vi "PolarNoGrid.vi"(0 "picture":picture, 5 "data array [mag, phase (deg)]":cluster{"magnitude":dbl, "phase":dbl}[](array[cluster]) {"phase" format="%0.2f"; "magnitude" format="%0.2f"}, 7 "top left point(0, 0)":cluster{"x":i16, "y":i16}, 9 "dimensions (w,h)":cluster{"width":i16, "height":i16}, 11 "polar attributes":T1={"maximum"=0.0, "minimum"=0.0, "clip to min"=FALSE, "log?(F)"=FALSE, "grid color"=6710886, "plot color"=65280, "fmt and prec"={"format"=enum."Decimal", "precision"=0}, "visible section"=8} {"minimum" format="%0.2f"; "maximum" format="%0.2f"}, 12 "Lines/Points":enum16{"Lines", "Points"}(ring), 13 "Size":u16=1) -> (4 "new picture":picture)   [LabVIEW 2014]
panel:
  in  "desired font(Application)":T2(ring)=enum."Application Font"
  in  "[user-specified font]":T3
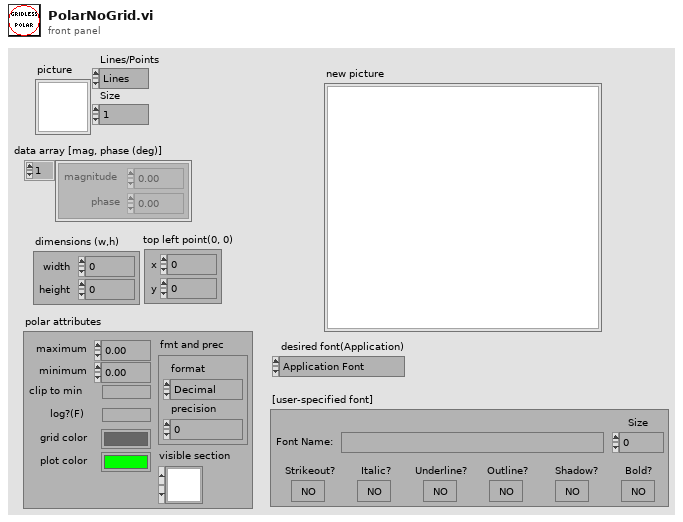
[diagram p1: front panel]
types:
  T1 = cluster{"maximum":dbl, "minimum":dbl, "clip to min":bool, "log?(F)":bool, "grid color":u32, "plot color":u32, "fmt and prec":cluster{"format":enum8{"Decimal", "Scientific", "Engineering", "Binary", "Octal", "Hex"}, "precision":u8}, "visible section":u16}
  T2 = enum16{"User-specified Font", "Application Font", "System Font", "Dialog Font"}
  T3 = cluster{"Font Name:":string, "Size":i16, "Strikeout?":bool, "Italic?":bool, "Underline?":bool, "Outline?":bool, "Shadow?":bool, "Bold?":bool}
  T4 = cluster{"left":i16, "top":i16, "right":i16, "bottom":i16}
  T5 = cluster{"pixel center":cluster{"x":i16, "y":i16}, "scale factors":cluster{"a":dbl, "b":dbl, "log?(F)":bool}, "grid color":u32, "start angle":dbl, "end angle":dbl, "tick length":i16, "pixel radius":i32}
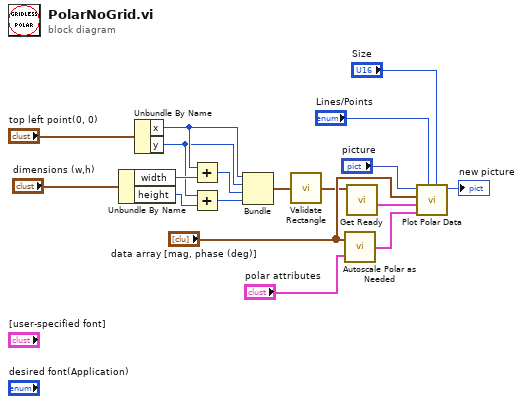
[diagram p0: block diagram]
diagram:
  n1 = Unbundle By Name("dimensions (w,h)") -> ("width"=w12:i16, "height"=w11:i16)
  n2 = Unbundle By Name("top left point(0, 0)") -> ("x"=w10:i16, "y"=w9:i16)
  n3 = Add(x=w10, y=w12) -> (x+y=w8:i16)
  n4 = Add(x=w9, y=w11) -> (x+y=w7:i16)
  n5 = Bundle("x"=w10, "y"=w9, w8, w7) -> (w6:cluster{"x":i16, "y":i16, i16, i16})  [unwired: 1 in]
  n6 = call <vilib>:"Validate Rectangle.vi"("rect"=w6) -> ("valid rect"=w3:T4)
  n7 = call <vilib>:"Autoscale Polar as Needed.vi"("polar attributes"="polar attributes", "data"="data array [mag, phase (deg)]") -> ("polar attributes"=w15:T1)
  n8 = call <vilib>:"Get Ready.vi"("rect"=w3) -> ("grid measurements"=w2:T5)  [unwired: 9 in, 1 out]
  n9 = call <vilib>:"Plot Polar Data.vi"("Size"="Size", "Lines/Points"="Lines/Points", "polar attributes"=w15, "grid measurements"=w2, "polar data"="data array [mag, phase (deg)]", "picture"="picture") -> ("new picture"=→"new picture":picture)  [unwired: 3 in]
